vi "Emit Data Count.vi"(8 "error in (no error)":errorcluster, 10 "Data Count":i32, 11 "Test 1 API in":refnum<class "Test 1.lvclass">) -> (0 "error out":errorcluster, 3 "Test 1 API out":refnum<class "Test 1.lvclass">)   [LabVIEW 2020, in "Scratchpad.lvlib" / "Test 1.lvlib" / "Test 1.lvclass"]
uses:
  Test 1/Test 1.lvclass
  C:/dev/lv20CE/relink/lv-artifex/Artifex/Actor/Actor.lvclass
  Artifex/Priority.ctl
  Artifex/Actor Proxy/Actor API.lvclass/Actor API.ctl
  Artifex/Actor Proxy/Emit Message.vi
  <vilib>/Utility/error.llb/Clear Errors.vi
  Data Count Msg/Data Count Msg.lvclass
  C:/dev/lv20CE/relink/lv-artifex/Artifex/Message/Message.lvclass
  Artifex/Priority Message Queue/Priority Enqueue.vi
  Artifex/Actor/Actor.lvclass
  Artifex/Artifex.lvlib
panel:
  in  "Priority (Normal)":T1=enum."Normal"
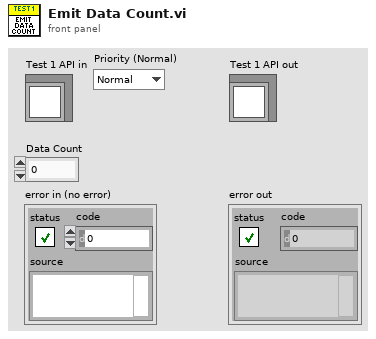
[diagram p1: front panel]
types:
  T1 = typedef "Artifex.lvlib/Priority.ctl" = enum16{"Low", "Normal", "High"}
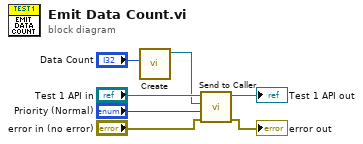
[diagram p0: block diagram]
diagram:
  n1 = call "Create.vi"("Data Count"="Data Count") -> ("Data Count Msg out"=w2:refnum<class "Data Count Msg.lvclass">)  [unwired: 9 in, 1 out]
  n2 = call "Send to Caller.vi"("error in (no error)"="error in (no error)", "Priority (Normal)"="Priority (Normal)", "Message"=w2, "Actor in"="Test 1 API in") -> ("error out"=→"error out":errorcluster, "Actor out"=→"Test 1 API out":refnum<class "Test 1.lvclass">)  [unwired: 6 in]
